vi "Get Sparse Marker Indexes [SM] Core.vi"(8 "error in (no error)":errorcluster, 9 "Marker Name (\"\")":string caption="marker name (\"\")", 10 "Indexes Array Size":i64 caption="indexes array size" format="%.0g", 11 "IVI_Fgen in":refnum<class "IVI_Fgen.lvclass">) -> (0 "error out":errorcluster, 1 "Indexes Array":i64[](array[numeric]) caption="indexes array", 2 "Indexes Actual Size":i64 caption="indexes actual size", 3 "IVI_Fgen out":refnum<class "IVI_Fgen.lvclass">)   [LabVIEW 2015, in "IVI_Fgen.lvlib" / "IVI_Fgen.lvclass"]
doc: "The VI returns the coerced indexes associated with the sparse marker. You can use the following VIs to specify indexes:\n\n- IviFgen Configure Sparse Marker [SM] VI\n- IviFgen Set Sparse Marker Indexes [SM] VI\n\nNote:\n\n(1) This VI is part of the IviFgenSparseMarker [SM] extension group."
uses:
  IVI_Fgen.lvclass
  IVI_Fgen.lvclass/IVI_Fgen.ctl
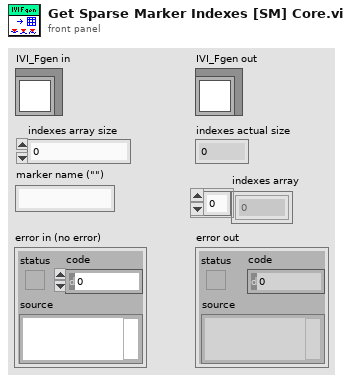
[diagram p1: front panel]
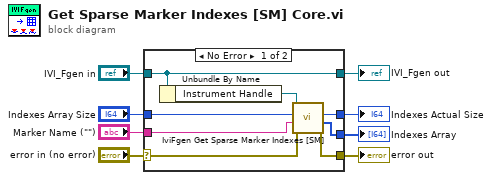
[diagram p0: block diagram]
diagram:
  n1 = case shown="No Error" "error in (no error)" {
    selector: "error in (no error)" -> [w14 w18]
    tunnel: [w13 w18] -> w7
    tunnel: [w16 w17] -> w5
    tunnel: "IVI_Fgen in" -> [w16 w17]
    tunnel: "Marker Name (\"\")" -> [w12 _]
    tunnel: "Indexes Array Size" -> [w11 _]
    tunnel: [w10 _] -> w2
    tunnel: [w9 _] -> w1
    frame No Error {
      n2 = Unbundle By Name(w16) -> ("Instrument Handle"=w15:refnum<k15>)
      n3 = call <vilib>:"IviFgen Get Sparse Marker Indexes [SM].vi"("error in (no error)"=w14, "Marker Name (\"\")"=w12, "Indexes Array Size"=w11, "instrument handle"=w15) -> ("error out"=w13:errorcluster, "Indexes Array"=w9:i64[], "Indexes Actural Size"=w10:i64)  [unwired: 4 in, 1 out]
    }
    frame Error {
    }
  }
  "error out" <- w7
  "IVI_Fgen out" <- w5
  "Indexes Actual Size" <- w2
  "Indexes Array" <- w1
